vi "RSNRPZ VI Tree.vi"   [LabVIEW 2017]
doc: "This instrument module provides programming support for the R&S NRP-Z Power Meter.\nThe VI Tree displays all the user-callable VIs of the instrument driver in an organized table.\n\nFor adetailed driver information including modification history, refer to the <B>RSNRPZ.chm </B>file."
panel:
  # "SEE DIAGRAM\nFOR VI TREE."
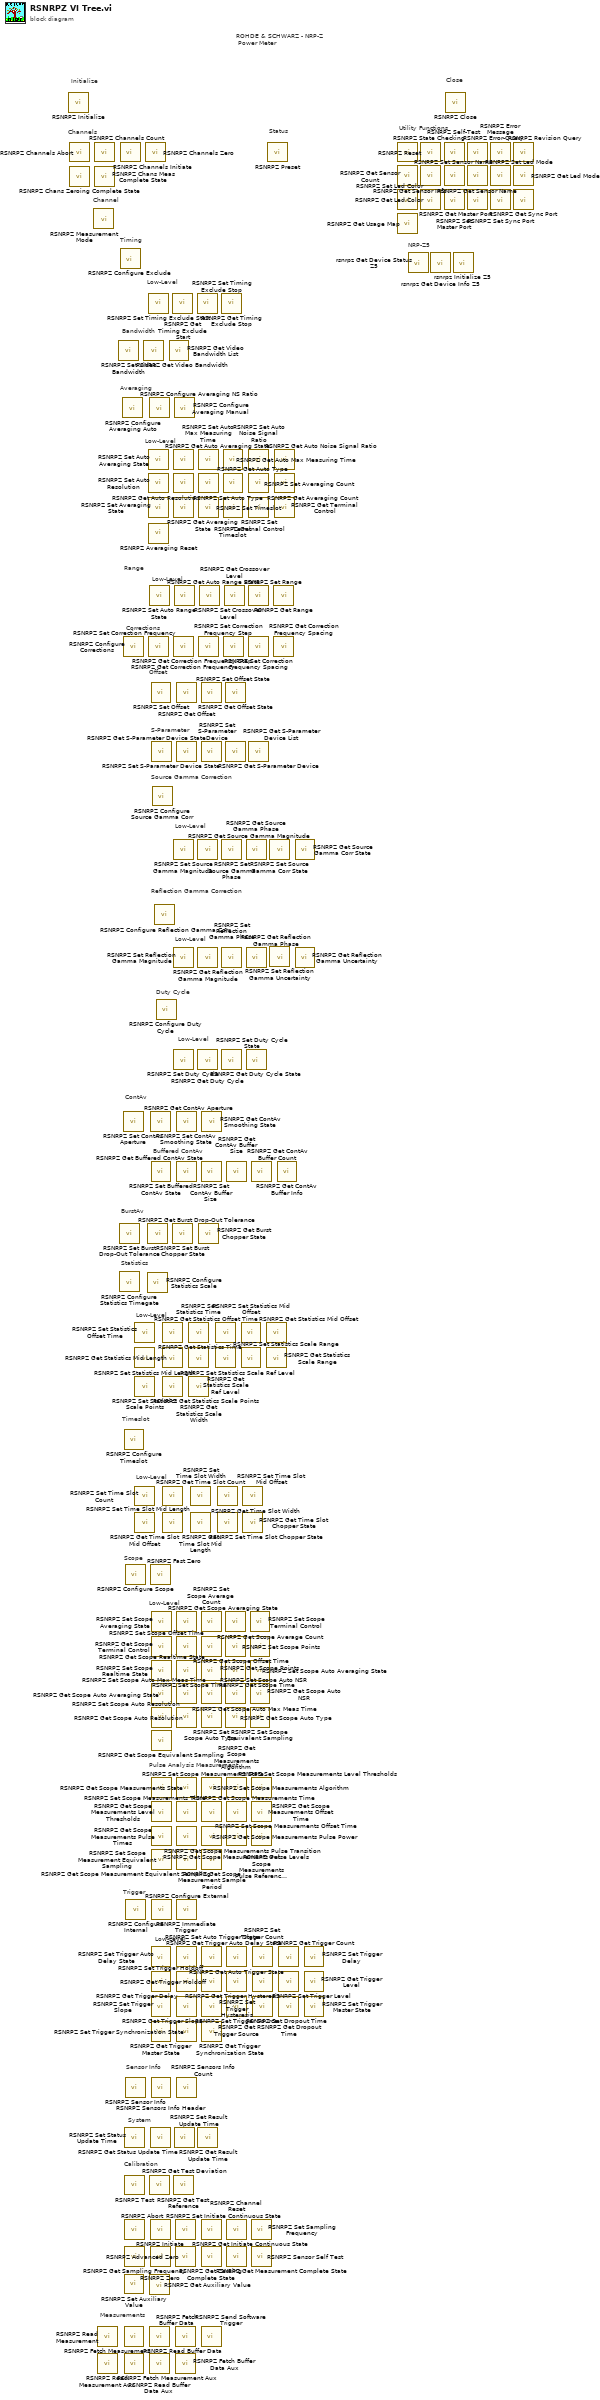
[diagram p0: block diagram]
diagram:
  # "NRP-Z5"
  # "Calibration"
  # "Pulse Analysis Measurement"
  # "System"
  # "Low-Level"
  # "Statistics"
  # "Bandwidth"
  # "Low-Level"
  # "Reflection Gamma Correction"
  # "Low-Level"
  # "Range"
  # "Utility Functions"
  # "Status"
  # "Measurements"
  # "Low-Level"
  # "Low-Level"
  # "Trigger"
  # "Sensor Info"
  # "Scope"
  # "Low-Level"
  # "Timeslot"
  # "Buffered ContAv"
  # "Low-Level"
  # "Low-Level"
  # "Duty Cycle"
  # "Source Gamma Correction"
  # "S-Parameter"
  # "Offset"
  # "Low-Level"
  # "Low-Level"
  # "BurstAv"
  # "ContAv"
  # "Corrections"
  # "Averaging"
  # "Timing"
  # "Channel"
  # "Channels"
  # "Close"
  # "Initialize"
  # "ROHDE & SCHWARZ - NRP-Z\n Power Meter"
  n1 = call <instrlib>:"RSNRPZ Initialize.vi"() -> ()  [unwired: 10 in, 2 out]
  n2 = call <instrlib>:"RSNRPZ Channels Abort.vi"() -> ()  [unwired: 10 in, 2 out]
  n3 = call <instrlib>:"RSNRPZ Chans Zeroing Complete State.vi"() -> ()  [unwired: 9 in, 3 out]
  n4 = call <instrlib>:"RSNRPZ Measurement Mode.vi"() -> ()  [unwired: 10 in, 2 out]
  n5 = call <instrlib>:"RSNRPZ Channels Count.vi"() -> ()  [unwired: 9 in, 3 out]
  n6 = call <instrlib>:"RSNRPZ Chans Meas Complete State.vi"() -> ()  [unwired: 9 in, 3 out]
  n7 = call <instrlib>:"RSNRPZ Read Measurement.vi"() -> ()  [unwired: 9 in, 3 out]
  n8 = call <instrlib>:"RSNRPZ Read Measurement Aux.vi"() -> ()  [unwired: 7 in, 5 out]
  n9 = call <instrlib>:"RSNRPZ Set Video Bandwidth.vi"() -> ()  [unwired: 10 in, 2 out]
  n10 = call <instrlib>:"RSNRPZ Set Burst Drop-Out Tolerance.vi"() -> ()  [unwired: 10 in, 2 out]
  n11 = call <instrlib>:"RSNRPZ Configure Statistics Timegate.vi"() -> ()  [unwired: 10 in, 2 out]
  n12 = call <instrlib>:"RSNRPZ Channels Initiate.vi"() -> ()  [unwired: 10 in, 2 out]
  n13 = call <instrlib>:"RSNRPZ Configure Exclude.vi"() -> ()  [unwired: 10 in, 2 out]
  n14 = call <instrlib>:"RSNRPZ Configure Averaging Auto.vi"() -> ()  [unwired: 10 in, 2 out]
  n15 = call <instrlib>:"RSNRPZ Configure Corrections.vi"() -> ()  [unwired: 14 in, 2 out]
  n16 = call <instrlib>:"RSNRPZ Set ContAv Aperture.vi"() -> ()  [unwired: 10 in, 2 out]
  n17 = call <instrlib>:"RSNRPZ Configure Timeslot.vi"() -> ()  [unwired: 10 in, 2 out]
  n18 = call <instrlib>:"RSNRPZ Set Auxiliary Value.vi"() -> ()  [unwired: 10 in, 2 out]
  n19 = call <instrlib>:"RSNRPZ Fetch Measurement.vi"() -> ()  [unwired: 9 in, 3 out]
  n20 = call <instrlib>:"RSNRPZ Fetch Measurement Aux.vi"() -> ()  [unwired: 7 in, 5 out]
  n21 = call <instrlib>:"RSNRPZ Set Status Update Time.vi"() -> ()  [unwired: 10 in, 2 out]
  n22 = call <instrlib>:"RSNRPZ Test.vi"() -> ()  [unwired: 9 in, 3 out]
  n23 = call <instrlib>:"RSNRPZ Abort.vi"() -> ()  [unwired: 10 in, 2 out]
  n24 = call <instrlib>:"RSNRPZ Get Sampling Frequency.vi"() -> ()  [unwired: 9 in, 3 out]
  n25 = call <instrlib>:"RSNRPZ Configure Scope.vi"() -> ()  [unwired: 14 in, 2 out]
  n26 = call <instrlib>:"RSNRPZ Sensor Info.vi"() -> ()  [unwired: 9 in, 3 out]
  n27 = call <instrlib>:"RSNRPZ Configure Internal.vi"() -> ()  [unwired: 10 in, 2 out]
  n28 = call <instrlib>:"RSNRPZ Set Statistics Offset Time.vi"() -> ()  [unwired: 10 in, 2 out]
  n29 = call <instrlib>:"RSNRPZ Set Statistics Mid Length.vi"() -> ()  [unwired: 10 in, 2 out]
  n30 = call <instrlib>:"RSNRPZ Set Statistics Scale Points.vi"() -> ()  [unwired: 10 in, 2 out]
  n31 = call <instrlib>:"RSNRPZ Set Time Slot Count.vi"() -> ()  [unwired: 10 in, 2 out]
  n32 = call <instrlib>:"RSNRPZ Get Time Slot Mid Offset.vi"() -> ()  [unwired: 9 in, 3 out]
  n33 = call <instrlib>:"RSNRPZ Get Video Bandwidth.vi"() -> ()  [unwired: 9 in, 3 out]
  n34 = call <instrlib>:"RSNRPZ Channels Zero.vi"() -> ()  [unwired: 10 in, 2 out]
  n35 = call <instrlib>:"RSNRPZ Configure Statistics Scale.vi"() -> ()  [unwired: 10 in, 2 out]
  n36 = call <instrlib>:"RSNRPZ Get Burst Drop-Out Tolerance.vi"() -> ()  [unwired: 9 in, 3 out]
  n37 = call <instrlib>:"RSNRPZ Set Timing Exclude Start.vi"() -> ()  [unwired: 10 in, 2 out]
  n38 = call <instrlib>:"RSNRPZ Set Auto Averaging State.vi"() -> ()  [unwired: 10 in, 2 out]
  n39 = call <instrlib>:"RSNRPZ Set Auto Resolution.vi"() -> ()  [unwired: 10 in, 2 out]
  n40 = call <instrlib>:"RSNRPZ Set Averaging State.vi"() -> ()  [unwired: 10 in, 2 out]
  n41 = call "RSNRPZ Averaging Reset.vi"() -> ()  [unwired: 10 in, 2 out]
  n42 = call <instrlib>:"RSNRPZ Set Correction Frequency.vi"() -> ()  [unwired: 10 in, 2 out]
  n43 = call <instrlib>:"RSNRPZ Configure Averaging NS Ratio.vi"() -> ()  [unwired: 10 in, 2 out]
  n44 = call <instrlib>:"RSNRPZ Set Auto Range State.vi"() -> ()  [unwired: 10 in, 2 out]
  n45 = call <instrlib>:"RSNRPZ Get Test Deviation.vi"() -> ()  [unwired: 9 in, 3 out]
  n46 = call <instrlib>:"RSNRPZ Get Auxiliary Value.vi"() -> ()  [unwired: 9 in, 3 out]
  n47 = call <instrlib>:"RSNRPZ Read Buffer Data.vi"() -> ()  [unwired: 8 in, 4 out]
  n48 = call <instrlib>:"RSNRPZ Read Buffer Data Aux.vi"() -> ()  [unwired: 6 in, 6 out]
  n49 = call <instrlib>:"RSNRPZ Get ContAv Aperture.vi"() -> ()  [unwired: 9 in, 3 out]
  n50 = call <instrlib>:"RSNRPZ Fast Zero.vi"() -> ()  [unwired: 10 in, 2 out]
  n51 = call <instrlib>:"RSNRPZ Get Status Update Time.vi"() -> ()  [unwired: 9 in, 3 out]
  n52 = call <instrlib>:"RSNRPZ Initiate.vi"() -> ()  [unwired: 10 in, 2 out]
  n53 = call <instrlib>:"RSNRPZ Zero.vi"() -> ()  [unwired: 10 in, 2 out]
  n54 = call <instrlib>:"RSNRPZ Set Offset.vi"() -> ()  [unwired: 10 in, 2 out]
  n55 = call <instrlib>:"RSNRPZ Set Buffered ContAv State.vi"() -> ()  [unwired: 10 in, 2 out]
  n56 = call <instrlib>:"RSNRPZ Set Trigger Auto Delay State.vi"() -> ()  [unwired: 10 in, 2 out]
  n57 = call <instrlib>:"RSNRPZ Get Trigger Delay.vi"() -> ()  [unwired: 9 in, 3 out]
  n58 = call <instrlib>:"RSNRPZ Set Trigger Slope.vi"() -> ()  [unwired: 10 in, 2 out]
  n59 = call <instrlib>:"RSNRPZ Get Trigger Master State.vi"() -> ()  [unwired: 9 in, 3 out]
  n60 = call <instrlib>:"RSNRPZ Sensors Info Header.vi"() -> ()  [unwired: 9 in, 3 out]
  n61 = call <instrlib>:"RSNRPZ Set S-Parameter Device State.vi"() -> ()  [unwired: 10 in, 2 out]
  n62 = call <instrlib>:"RSNRPZ Set Scope Averaging State.vi"() -> ()  [unwired: 10 in, 2 out]
  n63 = call <instrlib>:"RSNRPZ Get Scope Terminal Control.vi"() -> ()  [unwired: 9 in, 3 out]
  n64 = call <instrlib>:"RSNRPZ Set Scope Realtime State.vi"() -> ()  [unwired: 10 in, 2 out]
  n65 = call <instrlib>:"RSNRPZ Get Scope Auto Averaging State.vi"() -> ()  [unwired: 9 in, 3 out]
  n66 = call <instrlib>:"RSNRPZ Set Scope Auto Resolution.vi"() -> ()  [unwired: 10 in, 2 out]
  n67 = call <instrlib>:"RSNRPZ Get Scope Equivalent Sampling.vi"() -> ()  [unwired: 9 in, 3 out]
  n68 = call <instrlib>:"RSNRPZ Set Scope Measurements State.vi"() -> ()  [unwired: 10 in, 2 out]
  n69 = call <instrlib>:"RSNRPZ Get Scope Measurements Level Thresholds.vi"() -> ()  [unwired: 7 in, 5 out]
  n70 = call <instrlib>:"RSNRPZ Get Scope Measurements Pulse Times.vi"() -> ()  [unwired: 7 in, 5 out]
  n71 = call <instrlib>:"RSNRPZ Set Scope Measurement Equivalent Sampling.vi"() -> ()  [unwired: 10 in, 2 out]
  n72 = call <instrlib>:"RSNRPZ Configure External.vi"() -> ()  [unwired: 10 in, 2 out]
  n73 = call <instrlib>:"RSNRPZ Configure Source Gamma Corr.vi"() -> ()  [unwired: 10 in, 2 out]
  n74 = call <instrlib>:"RSNRPZ Configure Reflection Gamma Corr.vi"() -> ()  [unwired: 10 in, 2 out]
  n75 = call <instrlib>:"RSNRPZ Configure Duty Cycle.vi"() -> ()  [unwired: 14 in, 2 out]
  n76 = call <instrlib>:"RSNRPZ Get Statistics Offset Time.vi"() -> ()  [unwired: 9 in, 3 out]
  n77 = call <instrlib>:"RSNRPZ Get Statistics Mid Length.vi"() -> ()  [unwired: 9 in, 3 out]
  n78 = call <instrlib>:"RSNRPZ Get Statistics Scale Points.vi"() -> ()  [unwired: 9 in, 3 out]
  n79 = call <instrlib>:"RSNRPZ Get Time Slot Count.vi"() -> ()  [unwired: 9 in, 3 out]
  n80 = call <instrlib>:"RSNRPZ Set Time Slot Mid Length.vi"() -> ()  [unwired: 10 in, 2 out]
  n81 = call <instrlib>:"RSNRPZ Get Video Bandwidth List.vi"() -> ()  [unwired: 9 in, 3 out]
  n82 = call <instrlib>:"RSNRPZ Get Timing Exclude Start.vi"() -> ()  [unwired: 9 in, 3 out]
  n83 = call <instrlib>:"RSNRPZ Set Burst Chopper State.vi"() -> ()  [unwired: 10 in, 2 out]
  n84 = call "RSNRPZ Get Auto Averaging State.vi"() -> ()  [unwired: 9 in, 3 out]
  n85 = call <instrlib>:"RSNRPZ Get Auto Resolution.vi"() -> ()  [unwired: 9 in, 3 out]
  n86 = call <instrlib>:"RSNRPZ Get Averaging State.vi"() -> ()  [unwired: 9 in, 3 out]
  n87 = call <instrlib>:"RSNRPZ Get Correction Frequency.vi"() -> ()  [unwired: 9 in, 3 out]
  n88 = call <instrlib>:"RSNRPZ Set Source Gamma Magnitude.vi"() -> ()  [unwired: 10 in, 2 out]
  n89 = call <instrlib>:"RSNRPZ Set Reflection Gamma Magnitude.vi"() -> ()  [unwired: 10 in, 2 out]
  n90 = call <instrlib>:"RSNRPZ Set Duty Cycle.vi"() -> ()  [unwired: 10 in, 2 out]
  n91 = call <instrlib>:"RSNRPZ Get Test Reference.vi"() -> ()  [unwired: 9 in, 3 out]
  n92 = call <instrlib>:"RSNRPZ Configure Averaging Manual.vi"() -> ()  [unwired: 10 in, 2 out]
  n93 = call <instrlib>:"RSNRPZ Get Auto Range State.vi"() -> ()  [unwired: 9 in, 3 out]
  n94 = call <instrlib>:"RSNRPZ Set Result Update Time.vi"() -> ()  [unwired: 10 in, 2 out]
  n95 = call <instrlib>:"RSNRPZ Set Initiate Continuous State.vi"() -> ()  [unwired: 10 in, 2 out]
  n96 = call <instrlib>:"RSNRPZ Advanced Zero.vi"() -> ()  [unwired: 10 in, 2 out]
  n97 = call <instrlib>:"RSNRPZ Fetch Buffer Data.vi"() -> ()  [unwired: 8 in, 4 out]
  n98 = call <instrlib>:"RSNRPZ Fetch Buffer Data Aux.vi"() -> ()  [unwired: 6 in, 6 out]
  n99 = call <instrlib>:"RSNRPZ Set ContAv Smoothing State.vi"() -> ()  [unwired: 10 in, 2 out]
  n100 = call <instrlib>:"RSNRPZ Get Buffered ContAv State.vi"() -> ()  [unwired: 9 in, 3 out]
  n101 = call <instrlib>:"RSNRPZ Immediate Trigger.vi"() -> ()  [unwired: 10 in, 2 out]
  n102 = call <instrlib>:"RSNRPZ Get Trigger Auto Delay State.vi"() -> ()  [unwired: 9 in, 3 out]
  n103 = call <instrlib>:"RSNRPZ Set Trigger Holdoff.vi"() -> ()  [unwired: 10 in, 2 out]
  n104 = call <instrlib>:"RSNRPZ Get Trigger Slope.vi"() -> ()  [unwired: 9 in, 3 out]
  n105 = call <instrlib>:"RSNRPZ Set Trigger Synchronization State.vi"() -> ()  [unwired: 10 in, 2 out]
  n106 = call <instrlib>:"RSNRPZ Sensors Info Count.vi"() -> ()  [unwired: 9 in, 3 out]
  n107 = call <instrlib>:"RSNRPZ Get Offset.vi"() -> ()  [unwired: 9 in, 3 out]
  n108 = call <instrlib>:"RSNRPZ Get S-Parameter Device State.vi"() -> ()  [unwired: 9 in, 3 out]
  n109 = call <instrlib>:"RSNRPZ Get Scope Averaging State.vi"() -> ()  [unwired: 9 in, 3 out]
  n110 = call <instrlib>:"RSNRPZ Set Scope Offset Time.vi"() -> ()  [unwired: 10 in, 2 out]
  n111 = call <instrlib>:"RSNRPZ Get Scope Realtime State.vi"() -> ()  [unwired: 9 in, 3 out]
  n112 = call <instrlib>:"RSNRPZ Set Scope Auto Max Meas Time.vi"() -> ()  [unwired: 10 in, 2 out]
  n113 = call <instrlib>:"RSNRPZ Get Scope Auto Resolution.vi"() -> ()  [unwired: 9 in, 3 out]
  n114 = call <instrlib>:"RSNRPZ Get Scope Measurements State.vi"() -> ()  [unwired: 9 in, 3 out]
  n115 = call <instrlib>:"RSNRPZ Set Scope Measurements Time.vi"() -> ()  [unwired: 10 in, 2 out]
  n116 = call <instrlib>:"RSNRPZ Get Scope Measurements Pulse Transition.vi"() -> ()  [unwired: 7 in, 5 out]
  n117 = call <instrlib>:"RSNRPZ Get Scope Measurement Equivalent Sampling.vi"() -> ()  [unwired: 9 in, 3 out]
  n118 = call <instrlib>:"RSNRPZ Set Statistics Time.vi"() -> ()  [unwired: 10 in, 2 out]
  n119 = call <instrlib>:"RSNRPZ Set Statistics Scale Ref Level.vi"() -> ()  [unwired: 10 in, 2 out]
  n120 = call <instrlib>:"RSNRPZ Get Statistics Scale Width.vi"() -> ()  [unwired: 9 in, 3 out]
  n121 = call <instrlib>:"RSNRPZ Set Time Slot Width.vi"() -> ()  [unwired: 10 in, 2 out]
  n122 = call <instrlib>:"RSNRPZ Get Time Slot Mid Length.vi"() -> ()  [unwired: 9 in, 3 out]
  n123 = call <instrlib>:"RSNRPZ Set Timing Exclude Stop.vi"() -> ()  [unwired: 10 in, 2 out]
  n124 = call <instrlib>:"RSNRPZ Get Source Gamma Magnitude.vi"() -> ()  [unwired: 9 in, 3 out]
  n125 = call <instrlib>:"RSNRPZ Get Reflection Gamma Magnitude.vi"() -> ()  [unwired: 9 in, 3 out]
  n126 = call <instrlib>:"RSNRPZ Get Duty Cycle.vi"() -> ()  [unwired: 9 in, 3 out]
  n127 = call <instrlib>:"RSNRPZ Get Result Update Time.vi"() -> ()  [unwired: 9 in, 3 out]
  n128 = call <instrlib>:"RSNRPZ Set Auto Max Measuring Time.vi"() -> ()  [unwired: 10 in, 2 out]
  n129 = call <instrlib>:"RSNRPZ Set Auto Type.vi"() -> ()  [unwired: 10 in, 2 out]
  n130 = call <instrlib>:"RSNRPZ Set Timeslot.vi"() -> ()  [unwired: 10 in, 2 out]
  n131 = call <instrlib>:"RSNRPZ Set Correction Frequency Step.vi"() -> ()  [unwired: 10 in, 2 out]
  n132 = call <instrlib>:"RSNRPZ Get Burst Chopper State.vi"() -> ()  [unwired: 9 in, 3 out]
  n133 = call <instrlib>:"RSNRPZ Set Crossover Level.vi"() -> ()  [unwired: 10 in, 2 out]
  n134 = call <instrlib>:"RSNRPZ Set Offset State.vi"() -> ()  [unwired: 10 in, 2 out]
  n135 = call <instrlib>:"RSNRPZ Set S-Parameter Device.vi"() -> ()  [unwired: 10 in, 2 out]
  n136 = call <instrlib>:"RSNRPZ Set ContAv Buffer Size.vi"() -> ()  [unwired: 10 in, 2 out]
  n137 = call <instrlib>:"RSNRPZ Set Scope Average Count.vi"() -> ()  [unwired: 10 in, 2 out]
  n138 = call <instrlib>:"RSNRPZ Get Scope Offset Time.vi"() -> ()  [unwired: 9 in, 3 out]
  n139 = call <instrlib>:"RSNRPZ Set Scope Time.vi"() -> ()  [unwired: 10 in, 2 out]
  n140 = call <instrlib>:"RSNRPZ Get Scope Auto Max Meas Time.vi"() -> ()  [unwired: 9 in, 3 out]
  n141 = call <instrlib>:"RSNRPZ Set Scope Auto Type.vi"() -> ()  [unwired: 10 in, 2 out]
  n142 = call <instrlib>:"RSNRPZ Get Initiate Continuous State.vi"() -> ()  [unwired: 9 in, 3 out]
  n143 = call <instrlib>:"RSNRPZ Get Zeroing Complete State.vi"() -> ()  [unwired: 9 in, 3 out]
  n144 = call <instrlib>:"RSNRPZ Send Software Trigger.vi"() -> ()  [unwired: 10 in, 2 out]
  n145 = call <instrlib>:"RSNRPZ Get ContAv Smoothing State.vi"() -> ()  [unwired: 9 in, 3 out]
  n146 = call <instrlib>:"RSNRPZ Set Scope Measurements Algorithm.vi"() -> ()  [unwired: 10 in, 2 out]
  n147 = call <instrlib>:"RSNRPZ Get Scope Measurements Time.vi"() -> ()  [unwired: 9 in, 3 out]
  n148 = call <instrlib>:"RSNRPZ Get Scope Measurements Pulse Power.vi"() -> ()  [unwired: 7 in, 5 out]
  n149 = call <instrlib>:"RSNRPZ Get Scope Measurement Sample Period.vi"() -> ()  [unwired: 9 in, 3 out]
  n150 = call <instrlib>:"RSNRPZ Set Auto Trigger State.vi"() -> ()  [unwired: 10 in, 2 out]
  n151 = call <instrlib>:"RSNRPZ Get Trigger Holdoff.vi"() -> ()  [unwired: 9 in, 3 out]
  n152 = call <instrlib>:"RSNRPZ Set Trigger Source.vi"() -> ()  [unwired: 10 in, 2 out]
  n153 = call <instrlib>:"RSNRPZ Get Trigger Synchronization State.vi"() -> ()  [unwired: 9 in, 3 out]
  n154 = call <instrlib>:"RSNRPZ Get Statistics Time.vi"() -> ()  [unwired: 9 in, 3 out]
  n155 = call <instrlib>:"RSNRPZ Get Statistics Scale Ref Level.vi"() -> ()  [unwired: 9 in, 3 out]
  n156 = call <instrlib>:"RSNRPZ Get Time Slot Width.vi"() -> ()  [unwired: 9 in, 3 out]
  n157 = call <instrlib>:"RSNRPZ Set Time Slot Chopper State.vi"() -> ()  [unwired: 10 in, 2 out]
  n158 = call <instrlib>:"RSNRPZ Get Timing Exclude Stop.vi"() -> ()  [unwired: 9 in, 3 out]
  n159 = call <instrlib>:"RSNRPZ Set Source Gamma Phase.vi"() -> ()  [unwired: 10 in, 2 out]
  n160 = call <instrlib>:"RSNRPZ Set Reflection Gamma Phase.vi"() -> ()  [unwired: 10 in, 2 out]
  n161 = call <instrlib>:"RSNRPZ Set Duty Cycle State.vi"() -> ()  [unwired: 10 in, 2 out]
  n162 = call <instrlib>:"RSNRPZ Get Auto Max Measuring Time.vi"() -> ()  [unwired: 9 in, 3 out]
  n163 = call <instrlib>:"RSNRPZ Get Auto Type.vi"() -> ()  [unwired: 9 in, 3 out]
  n164 = call <instrlib>:"RSNRPZ Get Timeslot.vi"() -> ()  [unwired: 9 in, 3 out]
  n165 = call <instrlib>:"RSNRPZ Get Correction Frequency Step.vi"() -> ()  [unwired: 9 in, 3 out]
  n166 = call <instrlib>:"RSNRPZ Get Crossover Level.vi"() -> ()  [unwired: 9 in, 3 out]
  n167 = call <instrlib>:"RSNRPZ Get Offset State.vi"() -> ()  [unwired: 9 in, 3 out]
  n168 = call <instrlib>:"RSNRPZ Get S-Parameter Device.vi"() -> ()  [unwired: 9 in, 3 out]
  n169 = call <instrlib>:"RSNRPZ Get Scope Average Count.vi"() -> ()  [unwired: 9 in, 3 out]
  n170 = call <instrlib>:"RSNRPZ Set Scope Points.vi"() -> ()  [unwired: 10 in, 2 out]
  n171 = call <instrlib>:"RSNRPZ Get Scope Time.vi"() -> ()  [unwired: 9 in, 3 out]
  n172 = call <instrlib>:"RSNRPZ Set Scope Auto NSR.vi"() -> ()  [unwired: 10 in, 2 out]
  n173 = call <instrlib>:"RSNRPZ Get Scope Auto Type.vi"() -> ()  [unwired: 9 in, 3 out]
  n174 = call <instrlib>:"RSNRPZ Get ContAv Buffer Size.vi"() -> ()  [unwired: 9 in, 3 out]
  n175 = call <instrlib>:"RSNRPZ Get Scope Measurements Algorithm.vi"() -> ()  [unwired: 9 in, 3 out]
  n176 = call <instrlib>:"RSNRPZ Set Scope Measurements Offset Time.vi"() -> ()  [unwired: 10 in, 2 out]
  n177 = call <instrlib>:"RSNRPZ Get Scope Measurements Pulse Levels.vi"() -> ()  [unwired: 8 in, 4 out]
  n178 = call <instrlib>:"RSNRPZ Channel Reset.vi"() -> ()  [unwired: 10 in, 2 out]
  n179 = call <instrlib>:"RSNRPZ Get Measurement Complete State.vi"() -> ()  [unwired: 9 in, 3 out]
  n180 = call <instrlib>:"RSNRPZ Get Auto Trigger State.vi"() -> ()  [unwired: 9 in, 3 out]
  n181 = call <instrlib>:"RSNRPZ Set Trigger Hysteresis.vi"() -> ()  [unwired: 10 in, 2 out]
  n182 = call <instrlib>:"RSNRPZ Get Trigger Source.vi"() -> ()  [unwired: 9 in, 3 out]
  n183 = call <instrlib>:"RSNRPZ Set Statistics Mid Offset.vi"() -> ()  [unwired: 10 in, 2 out]
  n184 = call <instrlib>:"RSNRPZ Set Statistics Scale Range.vi"() -> ()  [unwired: 10 in, 2 out]
  n185 = call <instrlib>:"RSNRPZ Set Time Slot Mid Offset.vi"() -> ()  [unwired: 10 in, 2 out]
  n186 = call <instrlib>:"RSNRPZ Get Time Slot Chopper State.vi"() -> ()  [unwired: 9 in, 3 out]
  n187 = call <instrlib>:"RSNRPZ Get Source Gamma Phase.vi"() -> ()  [unwired: 9 in, 3 out]
  n188 = call <instrlib>:"RSNRPZ Get Reflection Gamma Phase.vi"() -> ()  [unwired: 9 in, 3 out]
  n189 = call <instrlib>:"RSNRPZ Get Duty Cycle State.vi"() -> ()  [unwired: 9 in, 3 out]
  n190 = call <instrlib>:"RSNRPZ Set Auto Noise Signal Ratio.vi"() -> ()  [unwired: 10 in, 2 out]
  n191 = call <instrlib>:"RSNRPZ Set Averaging Count.vi"() -> ()  [unwired: 10 in, 2 out]
  n192 = call <instrlib>:"RSNRPZ Set Terminal Control.vi"() -> ()  [unwired: 10 in, 2 out]
  n193 = call <instrlib>:"RSNRPZ Set Range.vi"() -> ()  [unwired: 10 in, 2 out]
  n194 = call <instrlib>:"RSNRPZ Set Correction Frequency Spacing.vi"() -> ()  [unwired: 10 in, 2 out]
  n195 = call <instrlib>:"RSNRPZ Get S-Parameter Device List.vi"() -> ()  [unwired: 9 in, 3 out]
  n196 = call <instrlib>:"RSNRPZ Set Scope Terminal Control.vi"() -> ()  [unwired: 10 in, 2 out]
  n197 = call <instrlib>:"RSNRPZ Get Scope Points.vi"() -> ()  [unwired: 9 in, 3 out]
  n198 = call <instrlib>:"RSNRPZ Set Scope Auto Averaging State.vi"() -> ()  [unwired: 10 in, 2 out]
  n199 = call <instrlib>:"RSNRPZ Get Scope Auto NSR.vi"() -> ()  [unwired: 9 in, 3 out]
  n200 = call <instrlib>:"RSNRPZ Set Scope Equivalent Sampling.vi"() -> ()  [unwired: 10 in, 2 out]
  n201 = call <instrlib>:"RSNRPZ Get ContAv Buffer Count.vi"() -> ()  [unwired: 9 in, 3 out]
  n202 = call <instrlib>:"RSNRPZ Set Scope Measurements Level Thresholds.vi"() -> ()  [unwired: 10 in, 2 out]
  n203 = call <instrlib>:"RSNRPZ Get Scope Measurements Offset Time.vi"() -> ()  [unwired: 9 in, 3 out]
  n204 = call <instrlib>:"RSNRPZ Get Scope Measurements Pulse Reference Levels.vi"() -> ()  [unwired: 7 in, 5 out]
  n205 = call <instrlib>:"RSNRPZ Set Sampling Frequency.vi"() -> ()  [unwired: 10 in, 2 out]
  n206 = call <instrlib>:"RSNRPZ Sensor Self Test.vi"() -> ()  [unwired: 9 in, 3 out]
  n207 = call <instrlib>:"RSNRPZ Set Trigger Count.vi"() -> ()  [unwired: 10 in, 2 out]
  n208 = call <instrlib>:"RSNRPZ Get Trigger Hysteresis.vi"() -> ()  [unwired: 9 in, 3 out]
  n209 = call <instrlib>:"RSNRPZ Set Dropout Time.vi"() -> ()  [unwired: 10 in, 2 out]
  n210 = call <instrlib>:"RSNRPZ Get Statistics Mid Offset.vi"() -> ()  [unwired: 9 in, 3 out]
  n211 = call <instrlib>:"RSNRPZ Get Statistics Scale Range.vi"() -> ()  [unwired: 9 in, 3 out]
  n212 = call <instrlib>:"RSNRPZ Preset.vi"() -> ()  [unwired: 10 in, 2 out]
  n213 = call <instrlib>:"RSNRPZ Set Source Gamma Corr State.vi"() -> ()  [unwired: 10 in, 2 out]
  n214 = call <instrlib>:"RSNRPZ Set Reflection Gamma Uncertainty.vi"() -> ()  [unwired: 10 in, 2 out]
  n215 = call <instrlib>:"RSNRPZ Get Range.vi"() -> ()  [unwired: 9 in, 3 out]
  n216 = call <instrlib>:"RSNRPZ Get Correction Frequency Spacing.vi"() -> ()  [unwired: 9 in, 3 out]
  n217 = call <instrlib>:"RSNRPZ Get Auto Noise Signal Ratio.vi"() -> ()  [unwired: 9 in, 3 out]
  n218 = call <instrlib>:"RSNRPZ Get Averaging Count.vi"() -> ()  [unwired: 9 in, 3 out]
  n219 = call <instrlib>:"RSNRPZ Get Terminal Control.vi"() -> ()  [unwired: 9 in, 3 out]
  n220 = call <instrlib>:"RSNRPZ Get ContAv Buffer Info.vi"() -> ()  [unwired: 9 in, 3 out]
  n221 = call <instrlib>:"RSNRPZ Get Trigger Count.vi"() -> ()  [unwired: 9 in, 3 out]
  n222 = call <instrlib>:"RSNRPZ Set Trigger Level.vi"() -> ()  [unwired: 10 in, 2 out]
  n223 = call <instrlib>:"RSNRPZ Get Dropout Time.vi"() -> ()  [unwired: 9 in, 3 out]
  n224 = call <instrlib>:"RSNRPZ Get Source Gamma Corr State.vi"() -> ()  [unwired: 9 in, 3 out]
  n225 = call <instrlib>:"RSNRPZ Get Reflection Gamma Uncertainty.vi"() -> ()  [unwired: 9 in, 3 out]
  n226 = call <instrlib>:"RSNRPZ Set Trigger Delay.vi"() -> ()  [unwired: 10 in, 2 out]
  n227 = call <instrlib>:"RSNRPZ Get Trigger Level.vi"() -> ()  [unwired: 9 in, 3 out]
  n228 = call <instrlib>:"RSNRPZ Set Trigger Master State.vi"() -> ()  [unwired: 10 in, 2 out]
  n229 = call <instrlib>:"RSNRPZ State Checking.vi"() -> ()  [unwired: 10 in, 2 out]
  n230 = call <instrlib>:"RSNRPZ Get Sensor Count.vi"() -> ()  [unwired: 10 in, 2 out]
  n231 = call <instrlib>:"RSNRPZ Set Led Color.vi"() -> ()  [unwired: 10 in, 2 out]
  n232 = call <instrlib>:"RSNRPZ Get Usage Map.vi"() -> ()  [unwired: 9 in, 3 out]
  n233 = call <instrlib>:"rsnrpz Get Device Status Z5.vi"() -> ()  [unwired: 9 in, 3 out]
  n234 = call <instrlib>:"RSNRPZ Reset.vi"() -> ()  [unwired: 10 in, 2 out]
  n235 = call <instrlib>:"RSNRPZ Get Sensor Info.vi"() -> ()  [unwired: 8 in, 4 out]
  n236 = call <instrlib>:"RSNRPZ Get Led Color.vi"() -> ()  [unwired: 9 in, 3 out]
  n237 = call <instrlib>:"rsnrpz Get Device Info Z5.vi"() -> ()  [unwired: 6 in, 6 out]
  n238 = call <instrlib>:"RSNRPZ Self-Test.vi"() -> ()  [unwired: 8 in, 4 out]
  n239 = call <instrlib>:"RSNRPZ Set Sensor Name.vi"() -> ()  [unwired: 10 in, 2 out]
  n240 = call <instrlib>:"RSNRPZ Set Master Port.vi"() -> ()  [unwired: 10 in, 2 out]
  n241 = call <instrlib>:"RSNRPZ Close.vi"() -> ()  [unwired: 11 in, 1 out]
  n242 = call <instrlib>:"rsnrpz Initialize Z5.vi"() -> ()  [unwired: 9 in, 3 out]
  n243 = call <instrlib>:"RSNRPZ Error-Query.vi"() -> ()  [unwired: 8 in, 4 out]
  n244 = call <instrlib>:"RSNRPZ Get Sensor Name.vi"() -> ()  [unwired: 9 in, 3 out]
  n245 = call <instrlib>:"RSNRPZ Get Master Port.vi"() -> ()  [unwired: 9 in, 3 out]
  n246 = call <instrlib>:"RSNRPZ Error Message.vi"() -> ()  [unwired: 9 in, 3 out]
  n247 = call <instrlib>:"RSNRPZ Set Led Mode.vi"() -> ()  [unwired: 10 in, 2 out]
  n248 = call <instrlib>:"RSNRPZ Set Sync Port.vi"() -> ()  [unwired: 10 in, 2 out]
  n249 = call <instrlib>:"RSNRPZ Revision Query.vi"() -> ()  [unwired: 8 in, 4 out]
  n250 = call <instrlib>:"RSNRPZ Get Led Mode.vi"() -> ()  [unwired: 9 in, 3 out]
  n251 = call <instrlib>:"RSNRPZ Get Sync Port.vi"() -> ()  [unwired: 9 in, 3 out]
